vi "removeTokenElement.vi"(7 "Endpoint Element Name":string, 8 "error in (no error)":errorcluster, 10 "Token element":T1, 11 "Oauth2 in":refnum<class "Oauth2.lvclass">) -> (0 "error out":errorcluster, 3 "Oauth2 out":refnum<class "Oauth2.lvclass">)   [LabVIEW 2017, in "Oauth2.lvclass"]
uses:
  Oauth2.lvclass
  OAuthToken/OAuth2 Token Element -- enum.ctl
  Oauth2.lvclass/Oauth2.ctl
  OAuthToken/OAuthAccessToken.lvclass
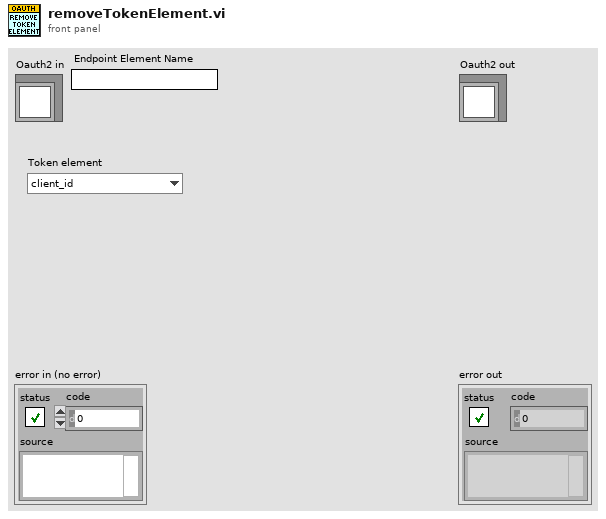
[diagram p1: front panel]
types:
  T1 = typedef "OAuthAccessToken.lvclass/OAuth2 Token Element -- enum.ctl" = enum16{"client_id", "client_secret", "response_type", "scope", "redirect_uri", "error", "error_description", "error_uri", "grant_type", "code", "access_token", "token_type", "expires_in", "username", "password", "refresh_token", "code_challenge", "code_challenge_method", "reverse_proxy_uri", "endpoint element", "access_type", "prompt", "id_token"}
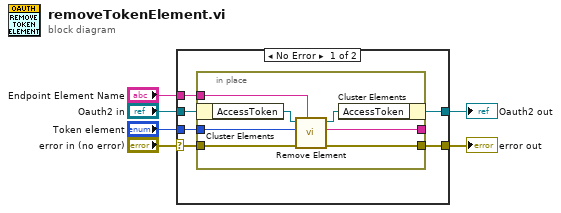
[diagram p0: block diagram]
diagram:
  n1 = case shown="No Error" "error in (no error)" {
    selector: "error in (no error)" -> [w10 w21]
    tunnel: [w9 w21] -> w5
    tunnel: [w7 w20] -> w3
    tunnel: "Oauth2 in" -> [w8 w20]
    tunnel: "Endpoint Element Name" -> [w12 _]
    tunnel: "Token element" -> [w11 _]
    frame No Error {
      n2 = in-place {
        in-place-border: w10 -> [w16]
        in-place-border: [w15] -> w9
        in-place-border: w11 -> [w17]
        in-place-border: w12 -> [w19]
        in-place-border: [w13] -> _
        n3 = in-place-cluster #1(w8) -> ("AccessToken"=w18:refnum<class "OAuthAccessToken.lvclass">)
        n4 = call "Remove Element.vi"("Endpoint element key"=w19, "error in (no error)"=w16, "Token element"=w17, "OAuthAccessToken in"=w18) -> ("error out"=w15:errorcluster, "Key"=w13:string, "OAuthAccessToken out"=w14:refnum<class "OAuthAccessToken.lvclass">)  [unwired: 5 in]
        n5 = in-place-cluster #1("AccessToken"=w14) -> (w7:refnum<class "Oauth2.lvclass">)
      }
    }
    frame Error {
    }
  }
  "error out" <- w5
  "Oauth2 out" <- w3
